vi "Generate Broken Board.vi"(1 "Assembly Line Input":T1) -> (0 "Assembly Line Input out":T1)   [LabVIEW 2023]
doc: "Generate a board image that will report a test failure in a correctly working system."
uses:
  Assembly Line Input.ctl
  Board Image.ctl
  Board Type Enum.ctl
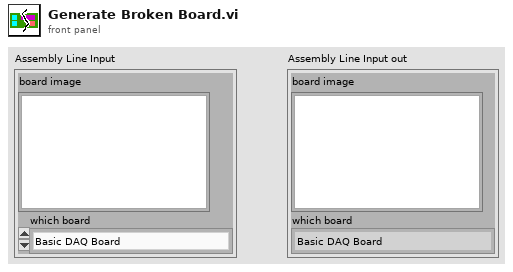
[diagram p1: front panel]
types:
  T1 = typedef "Assembly Line Input.ctl" = cluster{"board image":T2, "which board":T3}
  T2 = typedef "Board Image.ctl" = picture
  T3 = typedef "Board Type Enum.ctl" = enum16{"Basic DAQ Board", "Elite DAQ Board", "GPIB Board"}
  T4 = cluster{"left":i16, "top":i16, "right":i16, "bottom":i16}
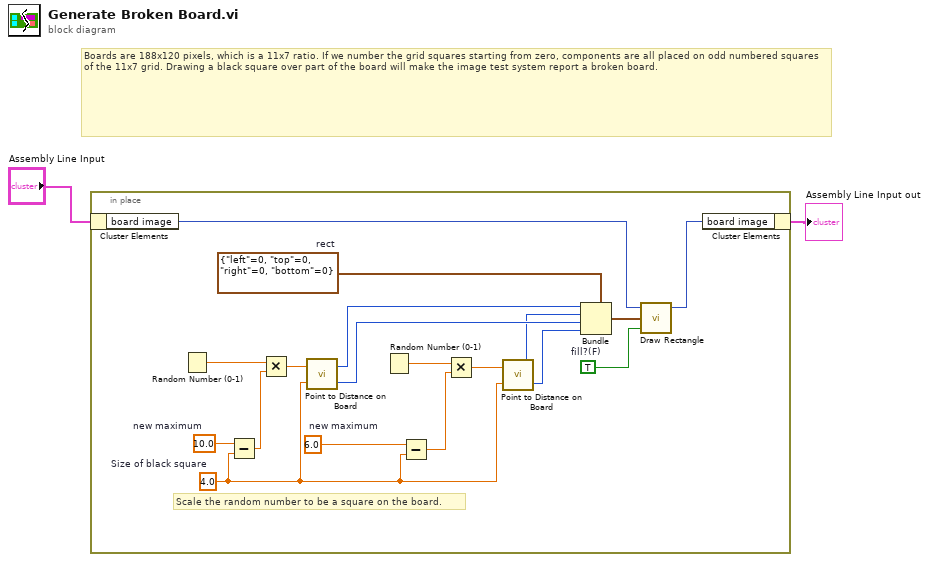
[diagram p0: block diagram]
diagram:
  # "Boards are 188x120 pixels, which is a 11x7 ratio. If we number the grid squares starting from zero, components are all placed on odd numbered squares of the 11x7 grid. Drawing a black square over part of the board will make the image test system report a broken board."
  n1 = in-place {
    w11 = 4.0  # Size of black square
    w14 = TRUE  # fill?(F)
    w20 = T4 {"left"=0, "top"=0, "right"=0, "bottom"=0}  # rect
    w13 = 10.0  # new maximum
    w12 = 6.0  # new maximum
    # "Scale the random number to be a square on the board."
    n2 = in-place-cluster #1("Assembly Line Input") -> ("board image"=w4:T2)
    n3 = Random Number (0-1)() -> (number: 0 to 1=w9:dbl)
    n4 = Subtract(x=w13, y=w11) -> (x-y=w8:dbl)
    n5 = Multiply(x=w9, y=w8) -> (x*y=w10:dbl)
    n6 = call "Point to Distance on Board.vi"("Size of square"=w11, "scaled value"=w10) -> ("end pixel"=w18:i16, "start pixel"=w19:i16)
    n7 = Random Number (0-1)() -> (number: 0 to 1=w7:dbl)
    n8 = Subtract(x=w12, y=w11) -> (x-y=w5:dbl)
    n9 = Multiply(x=w7, y=w5) -> (x*y=w6:dbl)
    n10 = call "Point to Distance on Board.vi"("Size of square"=w11, "scaled value"=w6) -> ("end pixel"=w16:i16, "start pixel"=w17:i16)
    n11 = Bundle(cluster=w20, "left"=w19, "top"=w17, "right"=w18, "bottom"=w16) -> (w15:T4)
    n12 = call <vilib>:"Draw Rectangle.vi"("picture"=w4, "rect"=w15, "fill?(F)"=w14) -> ("new picture"=w3:picture)  [unwired: 6 in]
    n13 = in-place-cluster #1("board image"=w3) -> (→"Assembly Line Input out":T1)
  }
